vi "DOE Search Program Name.vi"(11 "Program Name":string) -> (3 "LV Program":T1)   [LabVIEW 2016]
uses:
  Utility/Save File/File Setup (Public)/Type Definition/Save File DOE LabView Program.ctl
  Utility/Save File/File Setup.lvlib
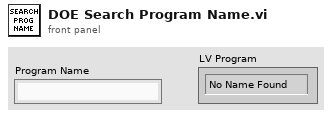
[diagram p1: front panel]
types:
  T1 = typedef "File Setup.lvlib/Save File DOE LabView Program.ctl" = enum16{"No Name Found", "DOE Stand", "Dishwasher Kitchen", "Portable Stand", "HEWH", "Dryer", "Dryer WILT", "HCC", "PRAT", "HEWH RLT", "Refrigeration", "Gas Water Heater"}
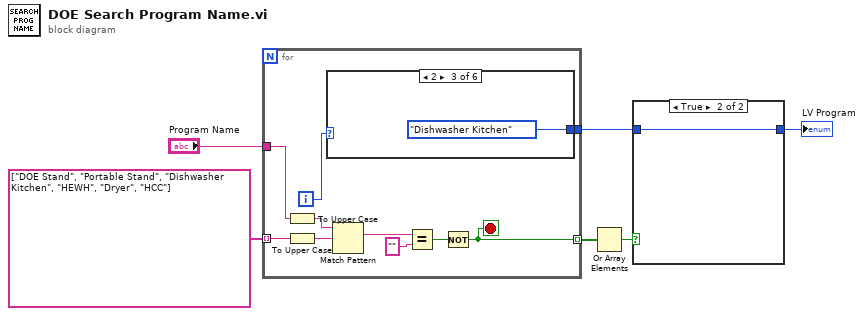
[diagram p0: block diagram]
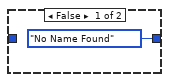
[diagram p2: hidden frame]
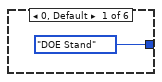
[diagram p3: hidden frame]
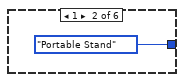
[diagram p4: hidden frame]
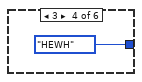
[diagram p5: hidden frame]
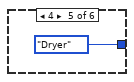
[diagram p6: hidden frame]
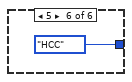
[diagram p7: hidden frame]
diagram:
  n1 = for {
    tunnel: string[] ["DOE Stand", "Portable Stand", "Dishwasher Kitchen", "HEWH", "Dryer", "HCC"] -> [w11] mode=indexing
    tunnel: "Program Name" -> [w13]
    tunnel: [w8] -> w1
    tunnel: [w7] -> w4 mode=indexing
    i -> [w9]
    stop <- w7 stop-if-true
    n2 = To Upper Case(1:w13) -> (0:w12:string)
    n3 = To Upper Case(1:w11) -> (0:w10:string)
    n4 = case shown="2" w9 {
      tunnel: [Save_File_DOE_LabView_Program."DOE Stand" ("LV Program") Save_File_DOE_LabView_Program."Portable Stand" ("LV Program") Save_File_DOE_LabView_Program."Dishwasher Kitchen" ("LV Program") Save_File_DOE_LabView_Program."HEWH" ("LV Program") Save_File_DOE_LabView_Program."Dryer" ("LV Program") Save_File_DOE_LabView_Program."HCC" ("LV Program")] -> w8
      frame 0, Default {
      }
      frame 1 {
      }
      frame 2 {
      }
      frame 3 {
      }
      frame 4 {
      }
      frame 5 {
      }
    }
    n5 = Match Pattern(string=w12, regular expression=w10) -> (match substring=w16:string)  [unwired: 1 in, 3 out]
    n6 = Equal?(x=w16, y="") -> (x = y?=w14:bool)
    n7 = Not(x=w14) -> (.not. x?=w7:bool)
  }
  n8 = Or Array Elements(Boolean array=w4) -> (logical OR=w3:bool)
  n9 = case shown="True" w3 {
    tunnel: [Save_File_DOE_LabView_Program."No Name Found" ("LV Program") w24] -> w2
    tunnel: w1 -> [_ w24]
    frame False {
    }
    frame True {
    }
  }
  "LV Program" <- w2
